vi "Format2DStringArray.vi"(1 "待格式化2D数组":string[][](array[string])) -> (0 "格式化2D数组":string[][](array[string]))   [LabVIEW 2019]
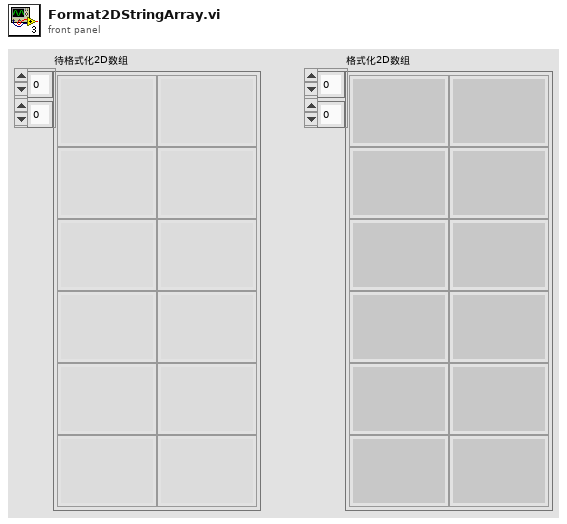
[diagram p1: front panel]
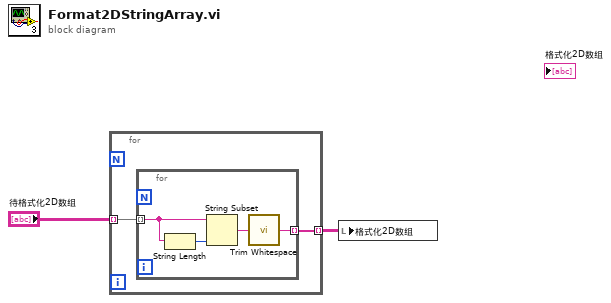
[diagram p0: block diagram]
diagram:
  n1 = for {
    tunnel: "待格式化2D数组" -> [w4] mode=indexing
    tunnel: [w3] -> w1 mode=indexing
    n2 = for {
      tunnel: w4 -> [w7] mode=indexing
      tunnel: [w8] -> w3 mode=indexing
      n3 = String Length(string=w7) -> (length=w5:i32)
      n4 = String Subset(string=w7, length (rest)=w5) -> (substring=w6:string)  [unwired: 1 in]
      n5 = call <vilib>:"Trim Whitespace.vi"("string"=w6) -> ("trimmed string"=w8:string)  [unwired: 1 in]
    }
  }
  n6 = local write "格式化2D数组"(w1) -> ()
